vi "GetWindowDisplayScale.vi"(8 "No Error":errorcluster, 11 "Window [SDL_Window *]":i64 format="%.0x") -> (0 "Error Out":errorcluster, 3 "Display Scale":sgl)   [LabVIEW 2026, in "SDL3.lvlib" / "Video.lvlib"]
doc: "<B>Summary</B>\nGet the content scale of a display.\n\n<B>Remarks</B>\nThe content scale is the expected scale for content based on the DPI settings of the display. For example, a 4K display might have a 2.0 (200%) display scale, which means that the user expects UI elements to be twice as big on this display, to aid in readability."
uses:
  Video.lvlib
  <vilib>/Utility/error.llb/Error Cluster From Error Code.vi
  Error/Error.lvlib
  Lib/SDL3.dll
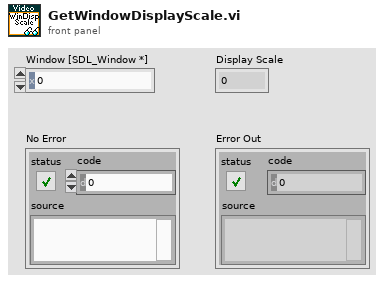
[diagram p1: front panel]
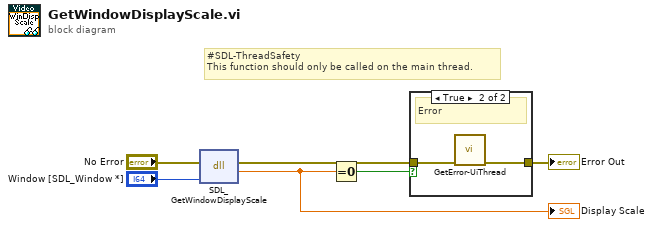
[diagram p0: block diagram]
diagram:
  # "#SDL-ThreadSafety\nThis function should only be called on the main thread."
  n1 = dll-call lib="C:/Users/saukko/Dev/LV-SDL3/Sources/SDL3/Lib/SDL3.*" fn="SDL_GetWindowDisplayScale"(error in="No Error", "window"="Window [SDL_Window *]") -> (error out=w2:errorcluster, "return type"=w3:sgl)  [unwired: 3 in, 1 out]
  "Display Scale" <- w3
  n2 = Equal To 0?(x=w3) -> (x = 0?=w1:bool)
  n3 = case shown="True" w1 {
    tunnel: w2 -> [w7 w9]
    tunnel: [w7 w8] -> w5
    frame False {
      # "Ok"
    }
    frame True {
      # "Error"
      n4 = call "GetError-UiThread.vi"("No Error"=w9) -> ("error out"=w8:errorcluster)  [unwired: 10 in]
    }
  }
  "Error Out" <- w5
